vi "Load Confluence Printer Settings.vi"(8 "Error in":errorcluster caption="Error in (no error)", 11 "Settings Path":path) -> (0 "Error out":errorcluster, 1 "Loaded Default?":bool, 3 "Confluence Printer Settings":T1={"Expand Structures"={"VI Member"={"By Folder Expand"=TRUE, "By Tree Expand"=TRUE, "By List Expand"=TRUE, "Methods Expand"=TRUE, "Controls Expand"=TRUE}, "Control Member"={"By Folder Expand"=TRUE, "By Tree Expand"=TRUE, "By List Expand"=TRUE, "Controls Expand"=TRUE}, "Interface"={"List Expand"=TRUE, "Controls Expand"=TRUE, "Methods Expand"=TRUE, "Inheritance Expand"=TRUE}, "Library"={"By Folder Expand"=TRUE, "By Tree Expand"=TRUE, "By List Expand"=TRUE, "Controls Expand"=TRUE, "Methods Expand"=TRUE, "Inheritance Expand"=TRUE}, "Class"={"By Folder Expand"=TRUE, "By Tree Expand"=TRUE, "By List Expand"=TRUE, "CPD Expand"=TRUE, "Controls Expand"=TRUE, "Methods Expand"=TRUE, "Set Accessors Expand"=TRUE, "Get Accessors Expand"=TRUE, "Inheritance Expand"=TRUE}}, "Sortable Tables"=TRUE, "Table Column Ordering"={"Class List"={"Minimal"=[], "Standard"=[], "Full"=[]}, "Library List"={"Minimal"=[], "Standard"=[], "Full"=[]}, "Control FP"={"Minimal"=[], "Standard"=[], "Full"=[]}, "Library Control Files"={"Minimal"=[], "Standard"=[], "Full"=[]}, "UI Methods"={"Minimal"=[], "Standard"=[], "Full"=[]}, "Method List"={"Minimal"=[], "Standard"=[], "Full"=[]}, "Interface Methods"={"Minimal"=[], "Standard"=[], "Full"=[]}, "LLB Methods"={"Minimal"=[], "Standard"=[], "Full"=[]}, "Library Methods"={"Minimal"=[], "Standard"=[], "Full"=[]}, "Class Methods"={"Minimal"=[], "Standard"=[], "Full"=[]}}})   [LabVIEW 2023, in "VIDoc Printer - Confluence.lvlib" / "VIDoc Settings - Confluence.lvclass"]
uses:
  VIDoc Settings - Confluence.lvclass
  VIDoc Settings/VIDoc Settings.lvclass
  ac5b38ed-98c3-46aa-8a0e-3b9f0d21d897.vi
  Confluence Printer Settings Cluster.ctl
  VI Info Column.ctl
  Control Info Column.ctl
  Class Info Column.ctl
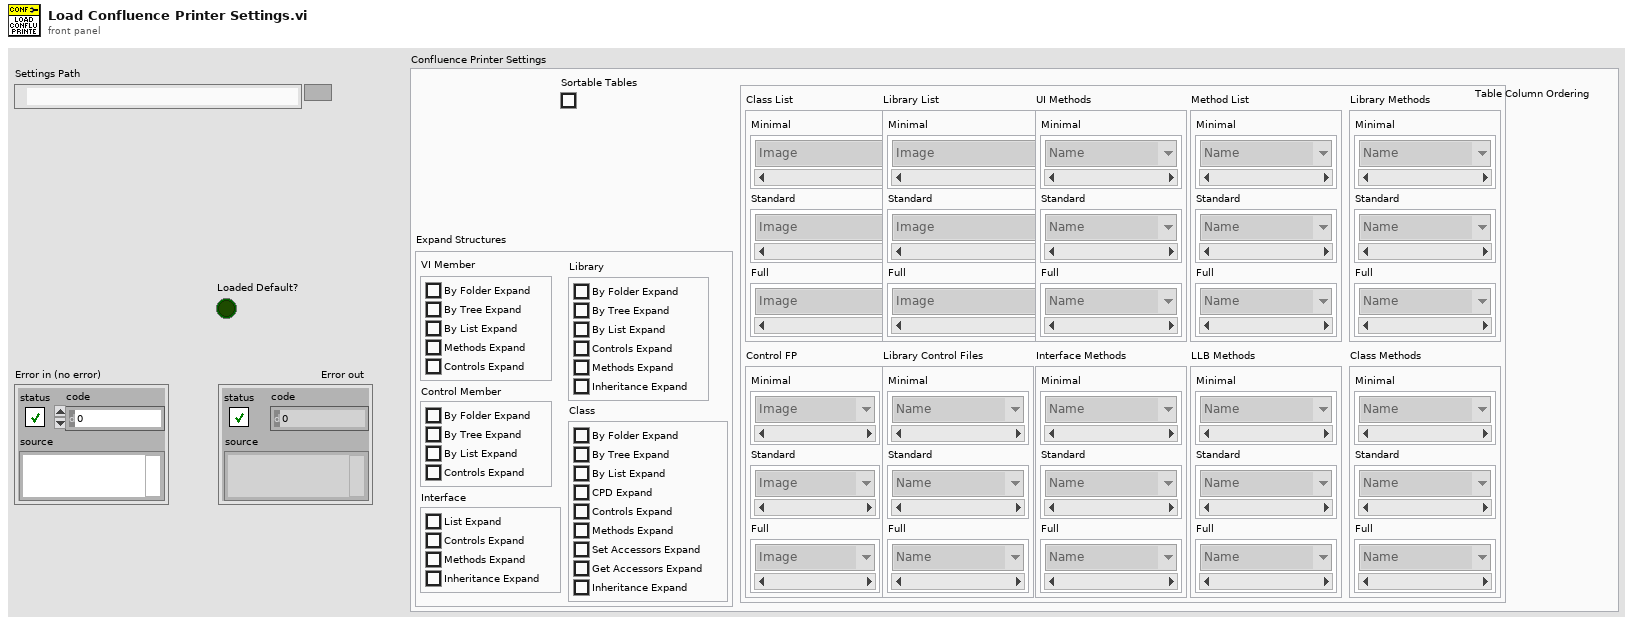
[diagram p1: front panel]
types:
  T1 = typedef "VIDoc Printer - Confluence.lvlib/VIDoc Settings - Confluence.lvclass/Confluence Printer Settings Cluster.ctl" = cluster{"Expand Structures":cluster{"VI Member":cluster{"By Folder Expand":bool, "By Tree Expand":bool, "By List Expand":bool, "Methods Expand":bool, "Controls Expand":bool}, "Control Member":cluster{"By Folder Expand":bool, "By Tree Expand":bool, "By List Expand":bool, "Controls Expand":bool}, "Interface":cluster{"List Expand":bool, "Controls Expand":bool, "Methods Expand":bool, "Inheritance Expand":bool}, "Library":cluster{"By Folder Expand":bool, "By Tree Expand":bool, "By List Expand":bool, "Controls Expand":bool, "Methods Expand":bool, "Inheritance Expand":bool}, "Class":cluster{"By Folder Expand":bool, "By Tree Expand":bool, "By List Expand":bool, "CPD Expand":bool, "Controls Expand":bool, "Methods Expand":bool, "Set Accessors Expand":bool, "Get Accessors Expand":bool, "Inheritance Expand":bool}}, "Sortable Tables":bool, "Table Column Ordering":cluster{"Class List":cluster{"Minimal":T2[], "Standard":T2[], "Full":T2[]}, "Library List":cluster{"Minimal":T2[], "Standard":T2[], "Full":T2[]}, "Control FP":cluster{"Minimal":T3[], "Standard":T3[], "Full":T3[]}, "Library Control Files":cluster{"Minimal":T4[], "Standard":T4[], "Full":T4[]}, "UI Methods":cluster{"Minimal":T4[], "Standard":T4[], "Full":T4[]}, "Method List":cluster{"Minimal":T4[], "Standard":T4[], "Full":T4[]}, "Interface Methods":cluster{"Minimal":T4[], "Standard":T4[], "Full":T4[]}, "LLB Methods":cluster{"Minimal":T4[], "Standard":T4[], "Full":T4[]}, "Library Methods":cluster{"Minimal":T4[], "Standard":T4[], "Full":T4[]}, "Class Methods":cluster{"Minimal":T4[], "Standard":T4[], "Full":T4[]}}}
  T2 = typedef "VIDoc Printer - Confluence.lvlib/VIDoc Settings - Confluence.lvclass/Class Info Column.ctl" = enum16{"Image", "Name", "Description", "Version", "Last Change", "Author", "Commit Hash", "Branch", "Qualified Name", "TransferMustOverrides", "ChildRefsRestricted"}
  T3 = typedef "VIDoc Printer - Confluence.lvlib/VIDoc Settings - Confluence.lvclass/Control Info Column.ctl" = enum16{"Image", "Name", "Description", "Caption", "Tip Strip", "Data Type", "Key Toggle"}
  T4 = typedef "VIDoc Printer - Confluence.lvlib/VIDoc Settings - Confluence.lvclass/VI Info Column.ctl" = enum16{"Name", "Conpane", "BD", "FP", "VI Icon", "Description", "Reentrant", "Inline", "Auto Error", "Compiled", "Code Complexity", "Data Size", "Debug", "Priority", "Rev", "Minimum Size", "Title", "FP Behavior", "FP Closeable", "Author", "Commit Hash", "Last Change", "Branch", "Scope", "Type", "Dispatch", "Must Override", "Must Use Parent", "Structure Tree"}
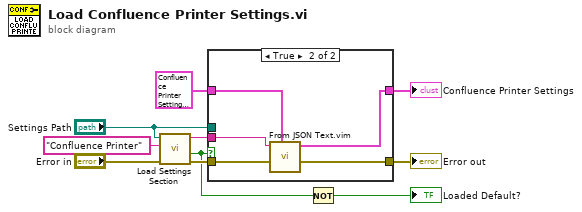
[diagram p0: block diagram]
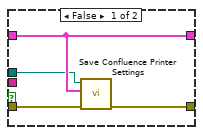
[diagram p2: hidden frame]
diagram:
  n1 = call "Load Settings Section.vi"("Error in"="Error in", "Section Name"="Confluence Printer", "JSON Settings Path"="Settings Path") -> ("Error out"=w8:errorcluster, "Found"=w2:bool, "JSON Object"=w7:string)  [unwired: 6 in]
  n2 = case shown="True" w2 {
    tunnel: w8 -> [w14 w19]
    tunnel: w7 -> [_ w18]
    tunnel: T1 {"Expand Structures"={"VI Member"={"By Folder Expand"=TRUE, "By Tree Expand"=TRUE, "By List Expand"=TRUE, "Methods Expand"=TRUE, "Controls Expand"=TRUE}, "Control Member"={"By Folder Expand"=TRUE, "By Tree Expand"=TRUE, "By List Expand"=TRUE, "Controls Expand"=TRUE}, "Interface"={"List Expand"=TRUE, "Controls Expand"=TRUE, "Methods Expand"=TRUE, "Inheritance Expand"=TRUE}, "Library"={"By Folder Expand"=TRUE, "By Tree Expand"=TRUE, "By List Expand"=TRUE, "Controls Expand"=TRUE, "Methods Expand"=TRUE, "Inheritance Expand"=TRUE}, "Class"={"By Folder Expand"=TRUE, "By Tree Expand"=TRUE, "By List Expand"=TRUE, "CPD Expand"=TRUE, "Controls Expand"=TRUE, "Methods Expand"=TRUE, "Set Accessors Expand"=TRUE, "Get Accessors Expand"=TRUE, "Inheritance Expand"=TRUE}}, "Sortable Tables"=TRUE, "Table Column Ordering"={"Class List"={"Minimal"=[], "Standard"=[], "Full"=[]}, "Library List"={"Minimal"=[], "Standard"=[], "Full"=[]}, "Control FP"={"Minimal"=[], "Standard"=[], "Full"=[]}, "Library Control Files"={"Minimal"=[], "Standard"=[], "Full"=[]}, "UI Methods"={"Minimal"=[], "Standard"=[], "Full"=[]}, "Method List"={"Minimal"=[], "Standard"=[], "Full"=[]}, "Interface Methods"={"Minimal"=[], "Standard"=[], "Full"=[]}, "LLB Methods"={"Minimal"=[], "Standard"=[], "Full"=[]}, "Library Methods"={"Minimal"=[], "Standard"=[], "Full"=[]}, "Class Methods"={"Minimal"=[], "Standard"=[], "Full"=[]}}} ("Confluence Printer Settings") -> [w12 w17]
    tunnel: [w12 w16] -> w5
    tunnel: [w13 w15] -> w4
    tunnel: "Settings Path" -> [w11 _]
    frame False {
      n3 = call "Save Confluence Printer Settings.vi"("Error in"=w14, "Confluence Printer Settings"=w12, "Settings Path"=w11) -> ("Error out"=w13:errorcluster)  [unwired: 8 in]
    }
    frame True {
      n4 = call "From JSON Text.vim"("Data Type and Default Value"=w17, "error in (no error)"=w19, "JSON"=w18) -> ("error out"=w15:errorcluster, "Data out"=w16:T1)  [unwired: 7 in]
    }
  }
  "Error out" <- w4
  "Confluence Printer Settings" <- w5
  n5 = Not(x=w2) -> (.not. x?=→"Loaded Default?":bool)
